vi "Golander pump 2 flows(mL per s, mL per rev).vi"(4 "State":i16=-1, 5 "Time":dbl format="%.2f", 6 "Sensor Values":dbl[](array[numeric]), 7 "Set Points":dbl[](array[numeric])=[12.0, 1.0, 1.0, 1.0]) -> (0 "required data":T4={"Set Point names"=["pump address", "on state 1 (167= states 1, 6, 7)", "on state 2 (23= states 2, 3)", "pump (mL/rev)", "flow 1 (mL/s)", "flow 2 (mL/s)"], "required number of setpoints"=6, "required number of sensors"=0, "Sensor names"=[]}, 3 "output value":dbl)   [LabVIEW 2019]
uses:
  pump 2 flows.ctl
  modbusrtu/MB ID-Address.ctl
  modbusrtu/SerialParameters.ctl
  modbusrtu/MB cmd buffer.ctl
panel:
  in  "MB ID-Address":T1
  in  "Pump cmds":T3
  # "failure at 80 ms"
  # "Enter the correct information for this control code in the required data structure below. Then make the current value default by right clicking on the border of the data structure. Select \"data operations\" and then select \"make current value default\". These values will be displayed by process controller."
  # "Mode: RTU\nAddresses: 1-247 (User Defined)\nBaud Rate: 9600\nData Bits: 8\nCRC: Even Parity\nStop Bit: 1"
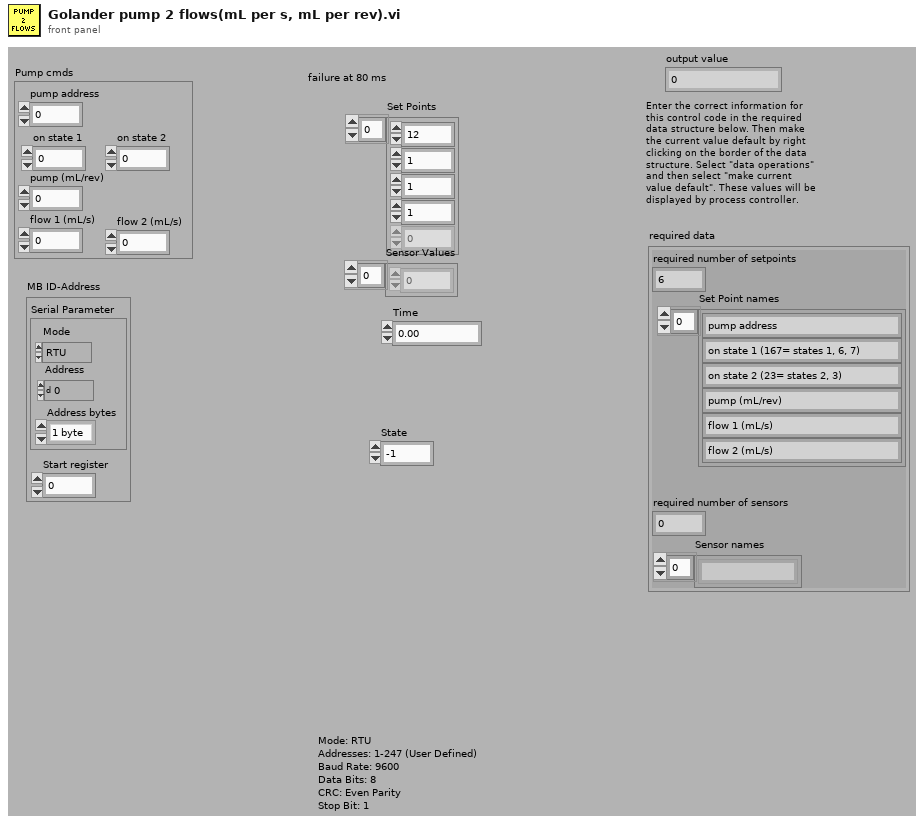
[diagram p1: front panel]
types:
  T1 = typedef "MB ID-Address.ctl" = cluster{"Serial Parameter":T2, "Start register":u16}
  T2 = typedef "SerialParameters.ctl" = cluster{"Mode":enum16{"RTU", "ASCII"}, "Address":u16, "Address bytes":enum16{"1 byte", "2 bytes"}}
  T3 = typedef "pump 2 flows.ctl" = cluster{"pump address":u8, "on state 1":i32, "on state 2":i32, "pump (mL/rev)":dbl, "flow 1 (mL/s)":dbl, "flow 2 (mL/s)":dbl}
  T4 = cluster{"Set Point names":string[], "required number of setpoints":u8, "required number of sensors":u8, "Sensor names":string[]}
  T5 = cluster{"Set Points[0]":dbl, "Set Points[1]":dbl, "Set Points[2]":dbl, "Set Points[3]":dbl, "Set Points[4]":dbl, "Set Points[5]":dbl}
  T6 = typedef "MB cmd buffer.ctl" = enum16{"ProCoDA", "MB succeed", "MB error", "MB Next Task", "ProCoDA read 1", "Commands pending"}
  T7 = typedef "MB status.ctl" = cluster{"ProCoDA Request":T8, "MB response":dbl[], "new cmd":bool, "error":errorcluster, "MB update(s)":dbl}
  T8 = typedef "ProCoDA MB Request.ctl" = cluster{"# registers":u8, "Data to write":u16[], "data interval (s)":dbl, "command":T9, "PC update (s)":dbl, "byte swap":T10, "data type":enum16{"float16", "int16"}}
  T9 = typedef "Read Write.ctl" = enum16{"Read", "Write"}
  T10 = typedef "byte swap.ctl" = enum16{"no swap", "swap registers"}
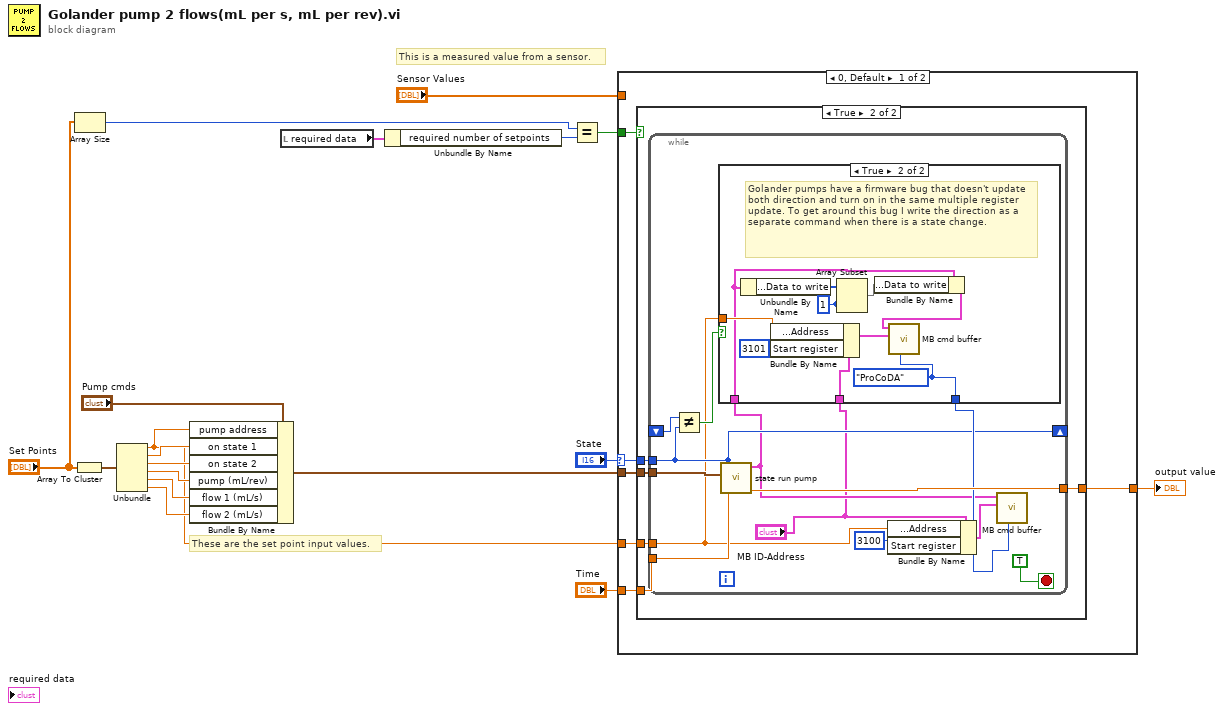
[diagram p0: block diagram]
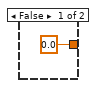
[diagram p2: hidden frame]
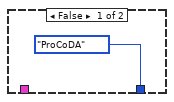
[diagram p3: hidden frame]
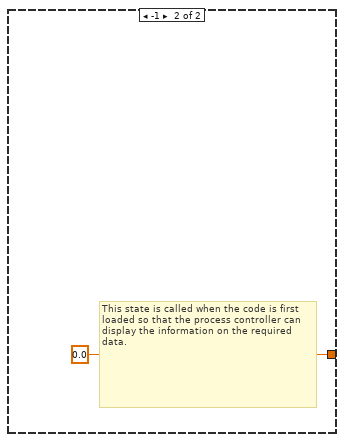
[diagram p4: hidden frame]
diagram:
  # "These are the set point input values."
  # "This is a measured value from a sensor."
  n1 = Array To Cluster(array="Set Points") -> (cluster=w16:T5)
  n2 = Array Size(array="Set Points") -> (size(s)=w6:i32)
  n3 = Unbundle(w16) -> ("Set Points[0]"=w1:dbl, "Set Points[1]"=w11:dbl, "Set Points[2]"=w10:dbl, "Set Points[3]"=w9:dbl, "Set Points[4]"=w8:dbl, "Set Points[5]"=w7:dbl)
  n4 = Bundle By Name(cluster="Pump cmds", "pump address"=w1, "on state 1"=w11, "on state 2"=w10, "pump (mL/rev)"=w9, "flow 1 (mL/s)"=w8, "flow 2 (mL/s)"=w7) -> (w15:T3)
  n5 = local read "required data"() -> (w3:T4)
  n6 = Unbundle By Name(w3) -> ("required number of setpoints"=w5:u8)
  n7 = Equal?(x=w6, y=w5) -> (x = y?=w4:bool)
  n8 = case shown="0, Default" "State" {
    selector: "State" -> [w21 _]
    tunnel: [w19 0.0 ("fraction on")] -> w13
    tunnel: w15 -> [w22 _]
    tunnel: "Sensor Values" -> [_ _]
    tunnel: "Time" -> [w23 _]
    tunnel: w4 -> [w24 _]
    tunnel: w1 -> [w20 _]
    frame 0, Default {
      n9 = case shown="True" w24 {
        tunnel: w22 -> [_ w30]
        tunnel: [0.0 ("rpm") w29] -> w19
        tunnel: w21 -> [_ w28]
        tunnel: w23 -> [_ w27]
        tunnel: w20 -> [_ w26]
        frame False {
        }
        frame True {
          n10 = while {
            tunnel: w30 -> [w42]
            tunnel: w28 -> [w36]
            tunnel: w27 -> [w38]
            tunnel: [w41] -> w29
            tunnel: w26 -> [w33]
            shift-right: [w36] -> _
            shift-left: _ -> [w35]
            stop <- TRUE stop-if-true
            n11 = Not Equal?(x=w35, y=w36) -> (x != y?=w34:bool)
            n12 = call "state run pump.vi"("Time"=w38, "pump command"=w42, "State"=w36) -> ("rpm"=w41:dbl, "MB status"=w32:T7)  [unwired: 1 in, 2 out]
            n13 = case shown="True" w34 {
              tunnel: "MB ID-Address" -> [_ w54]
              tunnel: w33 -> [_ w52]
              tunnel: [MB_cmd_buffer."ProCoDA" ("MB cmd buffer") w50] -> w37
              tunnel: w32 -> [_ w48]
              frame False {
              }
              frame True {
                w47 = 1 ("index")
                w50 = MB_cmd_buffer."ProCoDA" ("MB cmd buffer")
                # "Golander pumps have a firmware bug that doesn't update both direction and turn on in the same multiple register update. To get around this bug I write the direction as a separate command when there is a state change."
                n14 = Unbundle By Name(w48) -> ("ProCoDA Request.Data to write"=w45:u16[])
                n15 = Bundle By Name(cluster=w54, "Serial Parameter.Address"=w52, "Start register"=u16 3101 ("Register")) -> (w51:T1)
                n16 = Array Subset(array=w45, index=w47, length=w47) -> (w46:u16[])
                n17 = Bundle By Name(cluster=w48, "ProCoDA Request.Data to write"=w46) -> (w49:T7)
                n18 = call "MB cmd buffer.vi"("MB cmd buffer"=w50, "MB ID-Address in"=w51, "MB status in"=w49) -> ()  [unwired: 2 in, 7 out]
              }
            }
            n19 = Bundle By Name(cluster="MB ID-Address", "Serial Parameter.Address"=w33, "Start register"=u16 3100 ("MB ID-Address.Register")) -> (w40:T1)
            n20 = call "MB cmd buffer.vi"("MB cmd buffer"=w37, "MB ID-Address in"=w40, "MB status in"=w32) -> ()  [unwired: 2 in, 7 out]
          }
        }
      }
    }
    frame -1 {
      # "This state is called when the code is first loaded so that the process controller can display the information on the required data."
    }
  }
  "output value" <- w13
